vi "LWXPS_GroupMotionStatusGet.vi"(0 "XPS Reference IN":refnum<k24>, 5 "Group Name":string, 7 "Number of Positioners":i32, 11 "LabVIEW error IN":errorcluster) -> (4 "XPS Reference OUT":refnum<k24>, 6 "Returned error code":i32, 8 "Positioner Status":i32[](array[numeric]), 10 "XPS Error String":string, 15 "LabVIEW error OUT":errorcluster)   [LabVIEW 2014]
uses:
  D:/XPSQ8_LabView_Library/Development/Source/Dll/Newport.XPS.CommandInterface.dll
  Dll/Newport.XPS.CommandInterface.dll
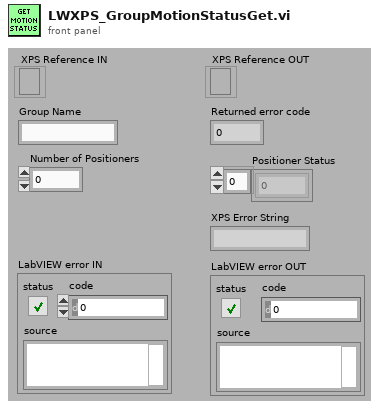
[diagram p1: front panel]
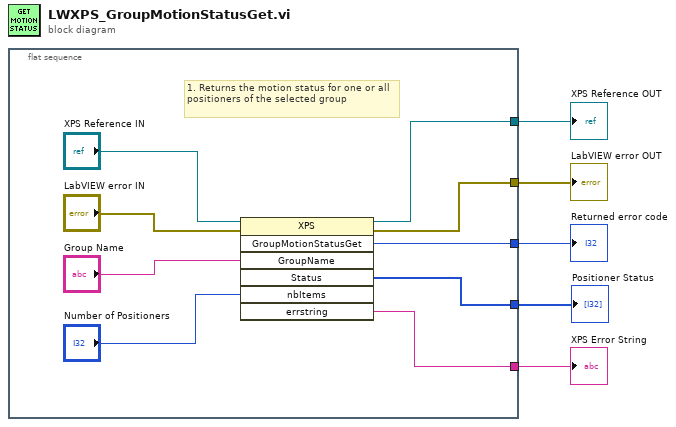
[diagram p0: block diagram]
diagram:
  n1 = flat-sequence {
    tunnel: [w12] -> w5
    tunnel: [w9] -> w4
    tunnel: [w13] -> w3
    tunnel: [w6] -> w2
    tunnel: [w8] -> w1
    frame #0 {
      # "1. Returns the motion status for one or all positioners of the selected group"
      n2 = invoke class="XPS" method="GroupMotionStatusGet"(reference="XPS Reference IN", error in="LabVIEW error IN", "GroupName"="Group Name", "nbItems"="Number of Positioners") -> (reference out=w12:refnum<k24>, error out=w9:errorcluster, "GroupMotionStatusGet"=w13:i32, "Status"=w8:i32[], "errstring"=w6:string)  [unwired: 3 in, 2 out]
    }
  }
  "XPS Reference OUT" <- w5
  "LabVIEW error OUT" <- w4
  "Returned error code" <- w3
  "XPS Error String" <- w2
  "Positioner Status" <- w1
